vi "Ref Plots Viewer.vi"() -> ()   [LabVIEW 2020]
uses:
  Typedefs/Ref plot graphs cluster.ctl
  RIG-SPECIFIC FILES/FPGA Refs/FPGA Ref.ctl
  Movement Correction/Typedefs/Reference plots window ctrl refs.ctl
  Typedefs/Save-Load enum.ctl
  Typedefs/Read Write Enum.ctl
  Global Variables/General Globals.vi
  Globals/gl_Windows Ctrl refs.vi
  <vilib>/Utility/error.llb/Error Cluster From Error Code.vi
  <vilib>/rvi/errors/niLvFpgaAdjustHostInterfaceError.vi
  <vilib>/rvi/interface/nirviReadWriteControl/nirviReadWriteControl.xnode
  <vilib>/rvi/interface/Simulation/niFpgaSimulationCallBeginRW.vi
  NiFpgaLv.dll
panel:
  out "Test GraphData Path":path
  in  "Append Date-Time":bool
  in  "Append file name":string
  out "MC Data Save ON":bool
  in  "Save MC Data":bool
  in  "Nth Frame":u16=11 min=10 step=10
  out "seen start":i16(graph)
  out "stop_bg":i16(graph)
  out "go_to_bg":i16(graph)
  out "MC":i16(graph)
  out "live_scan ind":i16(graph)
  out "start int":i16(graph)
  out "end of trial":i16(graph)
  out "bg mc Chart":i16(graph)
  in  "Frames":i16=1
  out "FPGA VI Reference Out":T1
  in  "Maximum Value":i32=4095
  in  "Minimum Value":i32
  out "Ref Image":T2(plugin-control)
  out "background_mc":bool
  out "bgsm_state":T3(ring)
  out "Acquire MC BG":bool
  out "rec_on_bg":bool
  out "aq state":T4(ring)
  in  "timed out?":bool
  in  "Acquisition completed":bool
  out "Protocol":string=" Last imaging type: None"
  out "Stop (ind)":bool
  out "error":errorcluster
  in  "Snapshot file path":path caption="Snapshot file path (data is appended if same file used)"
  in  "Buffer Size":i32=5000 min=5 max=10000 step=100
  in  "Refresh rate (ms)":u32=500 min=10 step=10
  in  "Snapshot":bool
  in  "Reset Graphs":bool
  out "Graphs cluster":T5
  # "(during live imaging)"
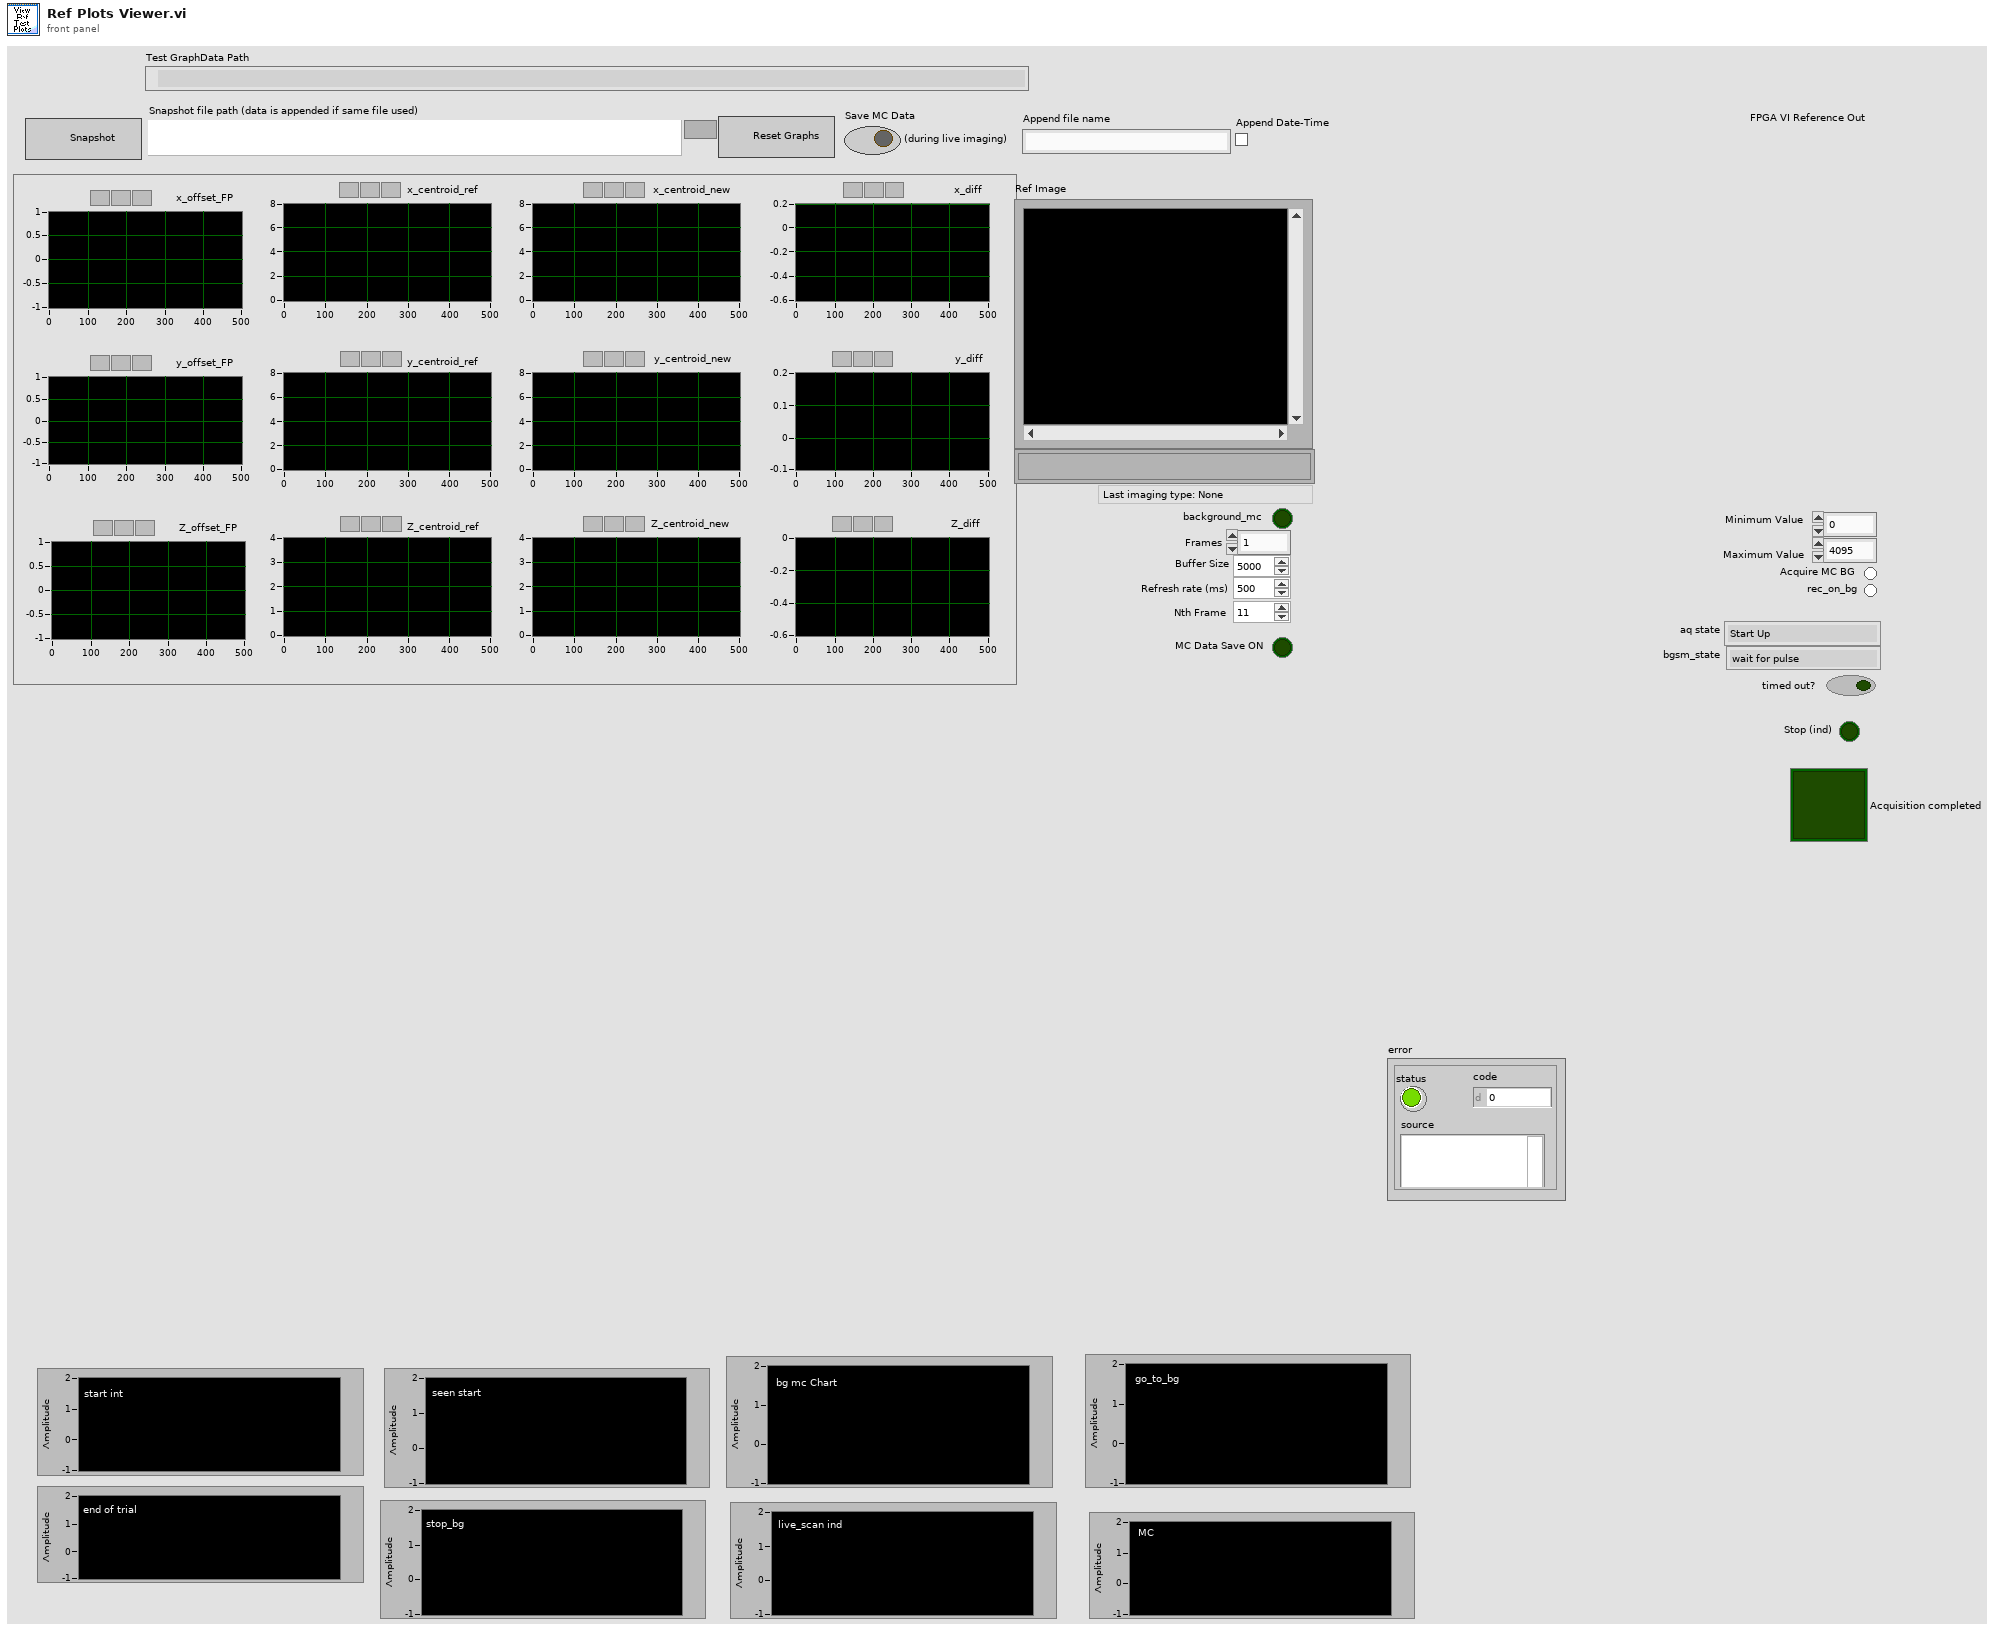
[diagram p1: front panel]
types:
  T1 = typedef "FPGA Ref.ctl" = refnum<k20>
  T2 = typedef "IMAQ Image.ctl" = refnum<image>
  T3 = enum16{"wait for pulse", "wiat for N after pulse", "refernce frame", "ref aod fill bg"}
  T4 = enum16{"Start Up", "Wait for Trigger", "Wait N after Trigger", "DAQ Pointing", "DAQ Scan", "Reference Scan", "Pointing AOL Fill", "Scan AOL FILL", "Reference AOL Fill"}
  T5 = typedef "Ref plot graphs cluster.ctl" = cluster{"x_offset_FP":dbl[], "y_offset_FP":dbl[], "x_centroid_ref":dbl[], "y_centroid_ref":dbl[], "x_centroid_new":dbl[], "y_centroid_new":dbl[], "x_diff":dbl[], "y_diff":dbl[], "Z_offset_FP":dbl[], "Z_centroid_ref":dbl[], "Z_centroid_new":dbl[], "Z_diff":dbl[]}
  T6 = typedef "Image Type" = u32
  T7 = typedef "Reference plots window ctrl refs.ctl" = cluster{"Refresh rate (ms)":refnum<vi>, "Buffer Size":refnum<vi>}
  T8 = typedef "Save-Load enum.ctl" = enum16{"Save to file", "Load from file", "Compare from file", "Save Backup"}
  T9 = enum16{"Obtain queue", "Call window", "Call & send signal", "Release queue"}
  T10 = typedef "Read Write Enum.ctl" = enum16{"Read", "Write"}
  T11 = typedef "AOL_Globals.ctl" = cluster{"Imaging Protocol":T12, "Number of POI":u16, "Number of Miniscans":u16, "Number of Trials":u16, "Number of Cycles ":u64, "# Averaged Frames":u16, "Laser power (%)":u8, "Pockels (V)":dbl, "Acquisition Length (sec)":dbl, "Fill time (us)":dbl, "POI Dwell time (us)":dbl, "Miniscan Dwell time per pixel (us)":dbl, "PMT 1":dbl, "PMT 2":dbl, "Back Apperture (mA)":dbl, "Frame Size":T13, "Center Frequency":dbl, "Field of View (norm)":dbl, "DwellTime (us)":dbl, "Wavelength (nm)":dbl, "Zoom":dbl, "AOL Z":dbl, "AOL Mode":T14, "GridXY":dbl, "GridZ":dbl, "TriggerPeriod (sec)":dbl, "Number of Pixels in Miniscan":u16, "Experiment folder path":path, "X centre":dbl, "Y centre":dbl, "Angle (degrees)":dbl, "Plane Mode":T15, "Threshold":u16[], "Regenerate Chirps":bool, "Rectangle ROI length (pixels)":u16, "Rectangle ROI height (pixels)":u16, "AOD fill":u16, "StartupDelay":i32, "Samples Wait after Trigger":u16, "Slip Cycle":u32, "Add Cycle":bool, "Functional Mode":T16, "Z Start":dbl, "Z Stop":dbl, "# Planes":i32, "Total Pixels":i32, "Variable Miniscan Pixels":u16[], "Use Variable Length":bool, "Use Variable Resolution":bool, "Laser power (%) at Z Start":u8, "Laser power (%) at Z Stop":u8, "Ref Z Step":i8, "Ref Dwell Time (us)":dbl, "Field of View (um)":dbl}
  T12 = typedef "Imaging Protocols enum.ctl" = enum16{"AOL Z-Stack", "Motor Z Stack", "Functional Acquisition", "Single Plane Acquisition", "Volume Acquisition", "Live Imaging", "Live Plane Imaging", "Live Volume Imaging"}
  T13 = typedef "Frame Size.ctl" = u16
  T14 = typedef "AOL modes.ctl" = enum16{"Raster", "Structural", "Pointing", "Mini Scan", "Alignment"}
  T15 = typedef "Plane Mode.ctl" = u16
  T16 = typedef "Functional Mode.ctl" = enum16{"Point", "Line", "Patch", "Plane", "Volume"}
  T17 = enum16{"Start Up", "Wait for Trigger", "Wait N after Trigger", "DAQ Pointing", "DAQ Scan", "Reference Scan", "Pointing AOL Fill", "Scan AOL FILL", "Reference AOL Fill", "galvo_moving"}
  T18 = cluster{"Conversion Method":u32, "Minimum Value":i32, "Maximum Value":i32, "Number Of Shifts":i32}
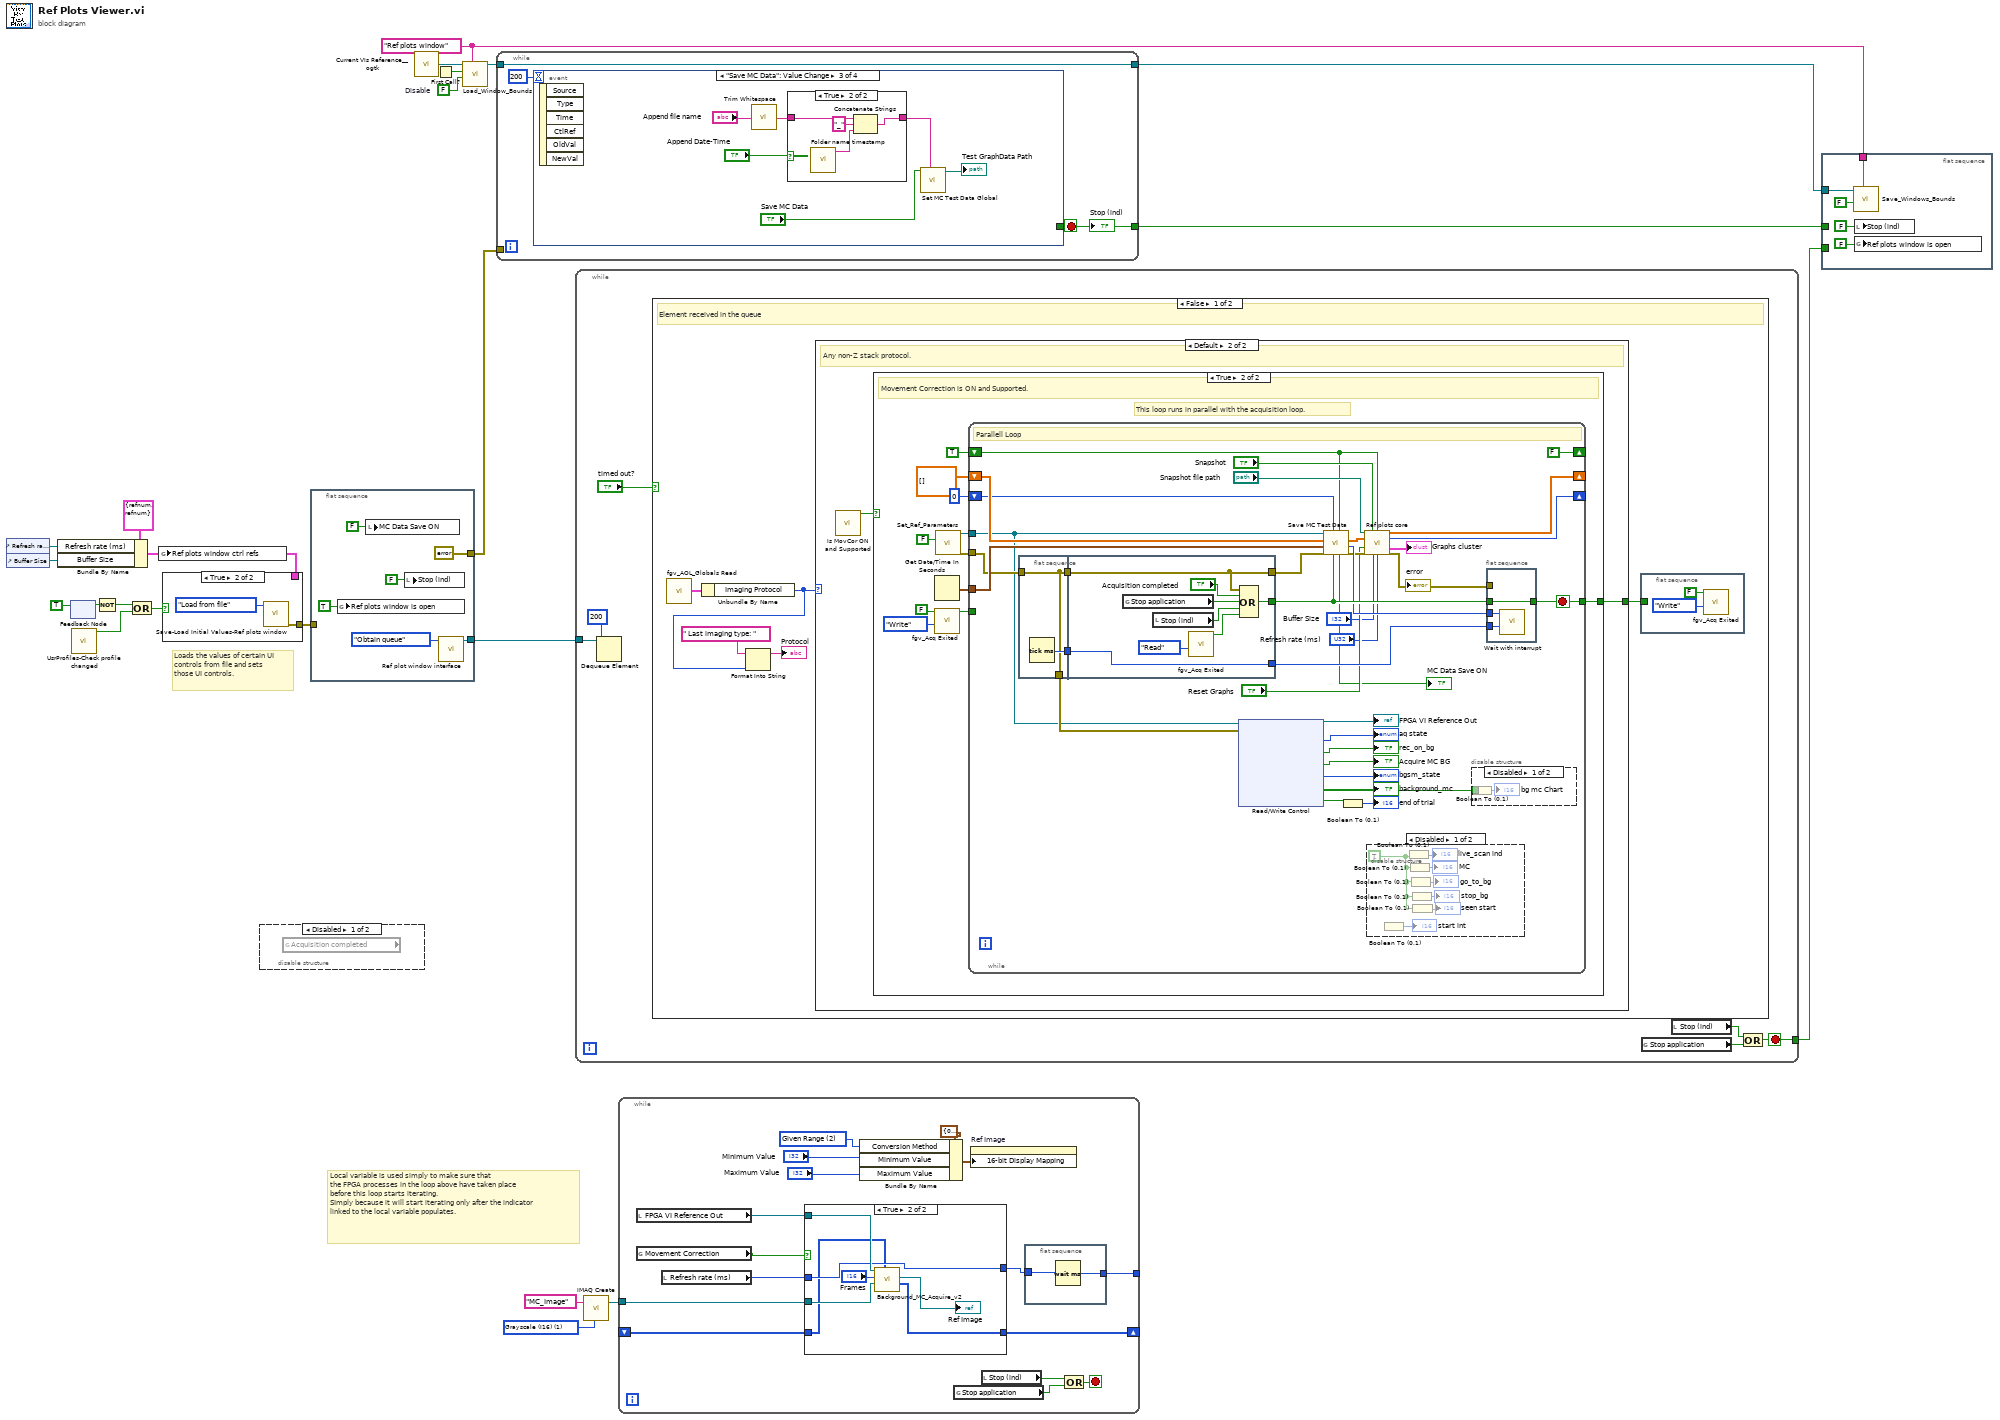
[diagram p0: block diagram]
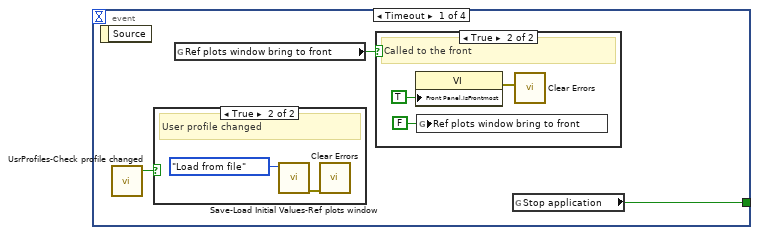
[diagram p5: hidden frame]
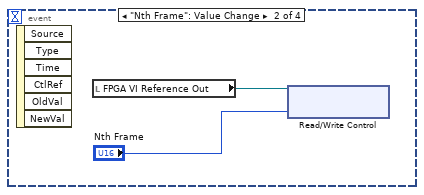
[diagram p8: hidden frame]
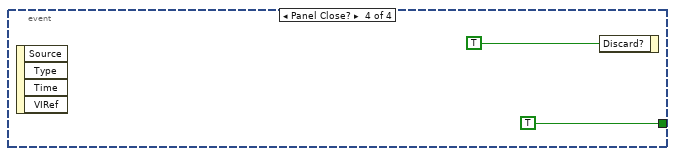
[diagram p10: hidden frame]
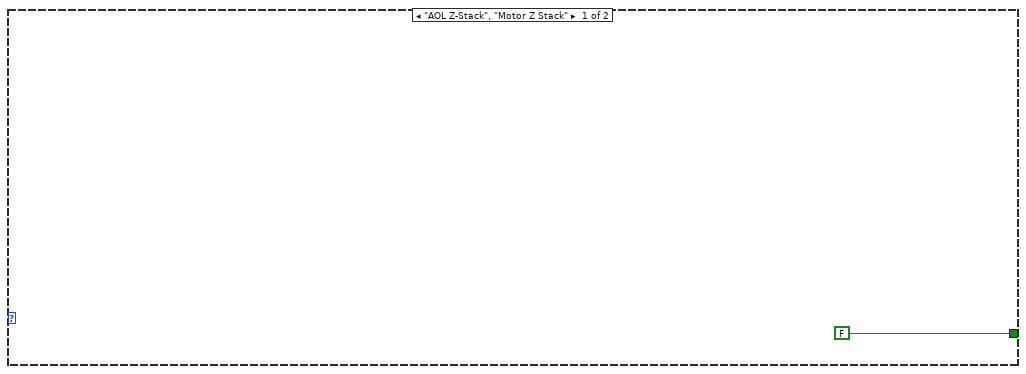
[diagram p11: hidden frame]
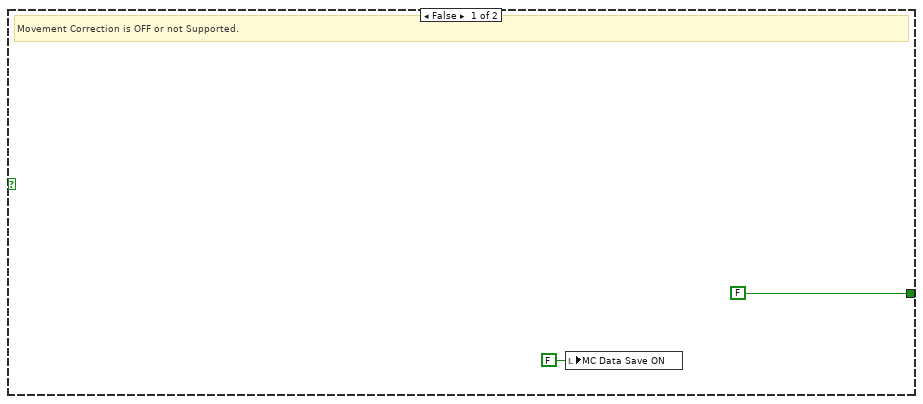
[diagram p12: hidden frame]
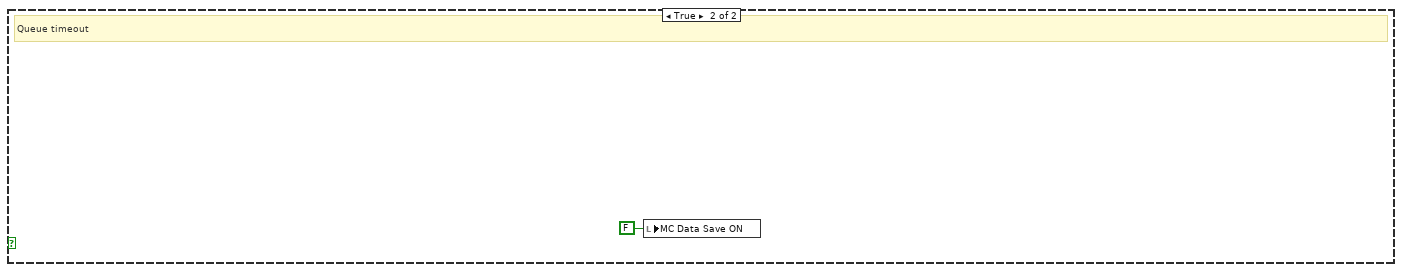
[diagram p15: hidden frame]
diagram:
  w2 = T6 1 items=["Grayscale (U8)", "Grayscale (I16)", "Grayscale (SGL)", "Complex (CSG)", "RGB (U32)", "HSL (U32)", "RGB (U64)", "Grayscale (U16)"] ("Image Type")
  w18 = FALSE  # Disable
  w6 = "Ref plots window" ("Window Name (i.e. Key)")
  # "Local variable is used simply to make sure that\nthe FPGA processes in the loop above have taken place\nbefore this loop starts iterating.\nSImply because it will start iterating only after the indicator\nlinked to the local variable populates."
  # "Loads the values of certain UI controls from file and sets those UI controls."
  n1 = control-ref of="Refresh rate (ms)"() -> (w13:refnum<vi>)
  n2 = control-ref of="Buffer Size"() -> (w12:refnum<vi>)
  n3 = Bundle By Name(cluster=T7 {"Refresh rate (ms)"=refnum, "Buffer Size"=refnum} ("Reference plots window ctrl refs"), "Refresh rate (ms)"=w13, "Buffer Size"=w12) -> (w14:T7)
  n4 = feedback #1() -> (w11:bool)  [unwired: 1 in]
  n5 = feedback-in #1(TRUE) -> ()
  n6 = call "UsrProfiles-Check profile changed.vi"() -> ("Profile changed"=w8:bool)  [unwired: 10 in, 1 out]
  n7 = Not(x=w11) -> (.not. x?=w9:bool)
  n8 = Compound Arithmetic op=OR(w9, w8) -> (w7:bool)
  n9 = global write "gl_Windows Ctrl refs.vi" "Ref plots window ctrl refs"(w14) -> ()
  n10 = case shown="True" w7 {
    tunnel: [_ w24] -> w16
    tunnel: w14 -> [_ _]
    frame False {
    }
    frame True {
      n11 = call "Save-Load Initial Values-Ref plots window.vi"("Function"=Save-Load_enum."Load from file") -> ("error out"=w24:errorcluster)  [unwired: 10 in]
    }
  }
  n12 = disable-structure shown="Disabled" {
    frame Disabled {
      n13 = global read "General Globals.vi" "Acquisition completed"() -> ()  [unwired: 1 out]
    }
    frame Enabled {
    }
  }
  n14 = flat-sequence {
    tunnel: [w30] -> w23
    tunnel: [errorcluster {"status"=FALSE, "code"=0, "source"=""} ("error out")] -> w21
    tunnel: w16 -> [_]
    frame #0 {
      n15 = global write "General Globals.vi" "Ref plots window is open"(TRUE ("Ref plots window is open")) -> ()
      n16 = local write "MC Data Save ON"(FALSE ("MC Data Save ON")) -> ()
      n17 = local write "Stop (ind)"(FALSE ("Stop (ind)")) -> ()
      n18 = call "Ref plot window interface.vi"("Function"=T9."Obtain queue") -> ("Ref plots window queue"=w30:refnum<queue>)  [unwired: 9 in, 1 out]
    }
  }
  n19 = call <userlib>:"Current VIs Reference__ogtk.vi"() -> ("Current VI's reference"=w20:refnum<vi>)  [unwired: 5 in]
  n20 = First Call?() -> (First Call?: T/F=w19:bool)
  n21 = call "Load_Window_Bounds.vi"("Window Name (i.e. Key)"=w6, "Disable"=w18, "First Call"=w19, "Window VI's Ref"=w20) -> ("reference out"=w17:refnum<vi>)  [unwired: 4 in, 3 out]
  n22 = while {
    tunnel: [w32] -> w4
    tunnel: w21 -> [_]
    tunnel: w17 -> [w33]
    tunnel: [w33] -> w5
    stop <- w32 stop-if-true
    n23 = event shown="[2] \"Save MC Data\": Value Change" {
      selector: _ -> [_ _ _ _]
      dyn-events: _ -> [_ _ _ _]
      timeout: 200 -> [_ _ _ _]
      tunnel: [w37 _ _ TRUE ("Stop application")] -> w32
      event Timeout {
        n24 = event-data() -> ()  [unwired: 1 in, 1 out]
        n25 = call "UsrProfiles-Check profile changed.vi"() -> ("Profile changed"=w35:bool)  [unwired: 10 in, 1 out]
        n26 = case shown="True" w35 {
          frame False {
            # "Idle"
          }
          frame True {
            # "User profile changed"
            n27 = call "Save-Load Initial Values-Ref plots window.vi"("Function"=Save-Load_enum."Load from file") -> ("error out"=w38:errorcluster)  [unwired: 10 in]
            n28 = call <vilib>:"Clear Errors.vi"("error in (no error)"=w38) -> ()  [unwired: 5 in, 2 out]
          }
        }
        n29 = global read "General Globals.vi" "Ref plots window bring to front"() -> (w36:bool)
        n30 = case shown="True" w36 {
          frame False {
            # "Idle"
          }
          frame True {
            # "Called to the front"
            n31 = property class="VI"("Front Panel.IsFrontmost"=TRUE ("Front Panel Window:Is Frontmost")) -> (error out=w41:errorcluster)  [unwired: 2 in, 1 out]
            n32 = global write "General Globals.vi" "Ref plots window bring to front"(FALSE ("\"Funct img\" bring to front")) -> ()
            n33 = call <vilib>:"Clear Errors.vi"("error in (no error)"=w41) -> ()  [unwired: 5 in, 2 out]
          }
        }
        n34 = global read "General Globals.vi" "Stop application"() -> (w37:bool)
      }
      event "Nth Frame": Value Change {
        n35 = event-data() -> ()  [unwired: 1 in, 6 out]
        n36 = local read "FPGA VI Reference Out"() -> (w44:T1)
        n37 = xnode "Read/Write Control"("FPGA VI Reference In"=w44, "ref_frame dilute"="Nth Frame") -> ()  [unwired: 1 in, 2 out]
      }
      event "Save MC Data": Value Change {
        n38 = event-data() -> ()  [unwired: 1 in, 6 out]
        n39 = call <vilib>:"Trim Whitespace.vi"("string"="Append file name") -> ("trimmed string"=w48:string)  [unwired: 1 in]
        n40 = case shown="True" "Append Date-Time" {
          tunnel: w48 -> [w51 w55]
          tunnel: [w51 w52] -> w47
          frame False {
          }
          frame True {
            n41 = call "Folder name timestamp.vi"() -> ("date/time string"=w53:string)  [unwired: 11 in]
            n42 = Concatenate Strings(w55, "_" ("string"), w53) -> (w52:string)
          }
        }
        n43 = call "Set MC Test Data Global.vi"("Append Name"=w47, "Save MC TestData"="Save MC Data") -> ("Test GraphData Path"=→"Test GraphData Path":path)  [unwired: 8 in, 1 out]
      }
      event Panel Close? {
        n44 = event-data() -> ()  [unwired: 1 in, 4 out]
        n45 = event-data("Discard?"=TRUE) -> ()  [unwired: 1 in, 1 out]
      }
    }
    "Stop (ind)" <- w32
  }
  n46 = while {
    tunnel: [w60] -> w22
    tunnel: w23 -> [w62]
    stop <- w60 stop-if-true
    n47 = Dequeue Element(queue=w62, timeout in ms (-1)=200) -> ()  [unwired: 1 in, 4 out]
    n48 = case shown="False" "timed out?" {
      frame False {
        # "Element received in the queue"
        n49 = call "fgv_AOL_Globals Read.vi"() -> ("AOL_Globals"=w67:T11)  [unwired: 9 in, 2 out]
        n50 = Unbundle By Name(w67) -> ("Imaging Protocol"=w66:T12)
        n51 = Format Into String(initial string=" Last imaging type: ", w66) -> (resulting string=→"Protocol":string)  [unwired: 2 in, 1 out]
        n52 = case shown="Default" w66 {
          tunnel: [FALSE w71] -> w68
          frame "AOL Z-Stack", "Motor Z Stack" {
          }
          frame Default {
            # "Any non-Z stack protocol."
            n53 = call "Is MovCor ON and Supported.vi"() -> ("MovCor is ON and Supported"=w70:bool)  [unwired: 11 in]
            n54 = case shown="True" w70 {
              tunnel: [FALSE w78] -> w71
              frame False {
                # "Movement Correction is OFF or not Supported."
                n55 = local write "MC Data Save ON"(FALSE ("MC Data Save ON")) -> ()
              }
              frame True {
                # "This loop runs in parallel with the acquisition loop."
                # "Movement Correction is ON and Supported."
                n56 = Get Date/Time In Seconds() -> (seconds since 1Jan1904=w80:timestamp)
                n57 = call "fgv_Acq Exited.vi"("Function"=Read_Write_Enum."Write", "Acquisition completed"=FALSE ("Timelapse?")) -> ("Acquisition completed"=w76:bool)  [unwired: 8 in, 1 out]
                n58 = call "Set_Ref_Parameters.vi"("use_increment_halfrate"=FALSE) -> ("error out"=w82:errorcluster, "FPGA VI Reference Out"=w81:T1)  [unwired: 8 in, 1 out]
                n59 = while {
                  tunnel: w81 -> [w90]
                  tunnel: w82 -> [w111]
                  shift-right: [w107] -> _
                  shift-left: dbl[][] [] -> [w117]
                  tunnel: w80 -> [w118]
                  shift-right: [FALSE] -> _
                  shift-left: TRUE -> [w96]
                  tunnel: [w116] -> w78
                  tunnel: w76 -> [_]
                  shift-right: [w106] -> _
                  shift-left: u32 0 ("Actual refresh rate (ms)") -> [w115]
                  stop <- w116 stop-if-true
                  # "Parallell Loop"
                  n60 = flat-sequence {
                    tunnel: [w130] -> w113
                    tunnel: [w129] -> w112
                    tunnel: w111 -> [w129]
                    tunnel: [w129] -> w91
                    tunnel: [w136] -> w109
                    tunnel: [w135] -> w114
                    tunnel: w113 -> [w135]
                    tunnel: w112 -> [w134]
                    tunnel: [w134] -> w110
                    frame #0 {
                      n61 = Tick Count (ms)() -> (millisecond timer value=w130:u32)
                    }
                    frame #1 {
                      n62 = global read "General Globals.vi" "Stop application"() -> (w138:bool)
                      n63 = local read "Stop (ind)"() -> (w132:bool)
                      n64 = call "fgv_Acq Exited.vi"("Function"=Read_Write_Enum."Read") -> ("Acquisition completed"=w133:bool)  [unwired: 9 in, 1 out]
                      n65 = Compound Arithmetic op=OR(w134, "Acquisition completed", w138, w132, w133) -> (w136:bool)
                    }
                  }
                  n66 = xnode ("Read/Write Control")("FPGA VI Reference In"=w90, "error in"=w91) -> ("FPGA VI Reference Out"=→"FPGA VI Reference Out":T1, "aq state"=→"aq state":T17, "rec_on_bg"=→"rec_on_bg":bool, "Acquire MC BG"=→"Acquire MC BG":bool, "bgsm_state"=→"bgsm_state":T3, "background_mc"=w88:bool, "end of trial"=w86:bool)  [unwired: 1 out]
                  "background_mc" <- w88
                  n67 = call "Save MC Test Data.vi"("Initialise"=w96, "Stop"=w109, "Actual refresh rate (ms)"=w115, "error in (no error)"=w110, "Initial Time Stamp"=w118, "Test Data In"=w117, "FPGA Ref in"=w90) -> ("error out"=w104:errorcluster, "MC state"=w108:enum16{"Waiting", "First frame", "Wrote Ref"}, "Test Data Out"=w97:dbl[][], "MC Data Save ON"=→"MC Data Save ON":bool)  [unwired: 1 in]
                  n68 = Boolean To (0,1)(Boolean=w86) -> (0, 1=→"end of trial":i16)
                  n69 = call "Ref plots core.vi"("Snapshot file path"="Snapshot file path", "Snapshot"="Snapshot", "Initialise"=w96, "Ref Test Data in in"=w97, "Reset Graphs"="Reset Graphs", "error in (no error)"=w104, "Buffer Size"="Buffer Size", "Refresh rate (ms)"="Refresh rate (ms)") -> ("Ref Test Data out"=w107:dbl[][], "Actual refresh rate (ms)"=w106:u32, "Graphs cluster"=→"Graphs cluster":T5, "error"=w105:errorcluster)  [unwired: 4 in]
                  "error" <- w105
                  n70 = disable-structure shown="Disabled" {
                    frame Disabled {
                      w121 = TRUE
                      n71 = Boolean To (0,1)() -> (0, 1=→"start int":i16)  [unwired: 1 in]
                      n72 = Boolean To (0,1)(Boolean=w121) -> (0, 1=→"live_scan ind":i16)
                      n73 = Boolean To (0,1)(Boolean=w121) -> (0, 1=→"MC":i16)
                      n74 = Boolean To (0,1)(Boolean=w121) -> (0, 1=→"go_to_bg":i16)
                      n75 = Boolean To (0,1)(Boolean=w121) -> (0, 1=→"stop_bg":i16)
                      n76 = Boolean To (0,1)(Boolean=w121) -> (0, 1=→"seen start":i16)
                    }
                    frame Enabled {
                    }
                  }
                  n77 = disable-structure shown="Disabled" {
                    disable-tunnel: w88 -> [w128 _]
                    frame Disabled {
                      n78 = Boolean To (0,1)(Boolean=w128) -> (0, 1=→"bg mc Chart":i16)
                    }
                    frame Enabled {
                    }
                  }
                  n79 = flat-sequence {
                    tunnel: w109 -> [w141]
                    tunnel: [w141] -> w116
                    tunnel: w114 -> [w140]
                    tunnel: w108 -> [w139]
                    tunnel: w105 -> [_]
                    frame #0 {
                      n80 = call "Wait with interrupt.vi"("Tick count at loop start (ms)"=w140, "Loop iteration (ms)"=w139) -> ()  [unwired: 10 in]
                    }
                  }
                }
              }
            }
          }
        }
        n81 = flat-sequence {
          tunnel: w68 -> [_]
          frame #0 {
            n82 = call "fgv_Acq Exited.vi"("Function"=Read_Write_Enum."Write", "Acquisition completed"=FALSE ("Timelapse?")) -> ()  [unwired: 8 in, 2 out]
          }
        }
      }
      frame True {
        # "Queue timeout"
        n83 = local write "MC Data Save ON"(FALSE ("MC Data Save ON")) -> ()
      }
    }
    n84 = global read "General Globals.vi" "Stop application"() -> (w63:bool)
    n85 = local read "Stop (ind)"() -> (w59:bool)
    n86 = Compound Arithmetic op=OR(w59, w63) -> (w60:bool)
  }
  n87 = call "IMAQ Create"("Image Name"="MC_Image", "Image Type"=w2) -> ("New Image"=w1:T2)  [unwired: 3 in, 1 out]
  n88 = while {
    tunnel: w1 -> [w157]
    tunnel: [w148] -> _
    shift-right: [w146] -> _
    shift-left: _ -> [w145]
    stop <- w158 stop-if-true
    w150 = u32 2 items=["Full Dynamic", "Downshift", "Given Range", "90% Dynamic", "Given Percent Range"] ("Conversion Method (Given Range)")
    n89 = local read "FPGA VI Reference Out"() -> (w156:T1)
    n90 = global read "General Globals.vi" "Movement Correction"() -> (w147:bool)
    n91 = local read "Refresh rate (ms)"() -> (w155:u32)
    n92 = case shown="True" w147 {
      tunnel: w156 -> [_ w171]
      tunnel: w157 -> [_ w170]
      tunnel: w155 -> [w164 w167]
      tunnel: [w164 w167] -> w149
      tunnel: [w163 w166] -> w146
      tunnel: w145 -> [w163 w165]
      frame False {
      }
      frame True {
        n93 = call "Background_MC_Acquire_v2.vi"("prev deleted portion"=w165, "Image In"=w170, "Frames"="Frames", "FPGA VI Reference In"=w171) -> ("deleted portion"=w166:u16[], "Image"=→"Ref Image":T2)  [unwired: 4 in, 2 out]
      }
    }
    n94 = Bundle By Name(cluster=T18 {"Conversion Method"=0, "Minimum Value"=0, "Maximum Value"=0, "Number Of Shifts"=0} ("16-bit Display Mapping:All Elements"), "Conversion Method"=w150, "Minimum Value"="Minimum Value", "Maximum Value"="Maximum Value") -> (w152:T18)
    n95 = global read "General Globals.vi" "Stop application"() -> (w159:bool)
    n96 = property on="Ref Image" class="ImageControl"("16-bit Display Mapping"=w152) -> ()  [unwired: 2 in, 2 out]
    n97 = local read "Stop (ind)"() -> (w160:bool)
    n98 = flat-sequence {
      tunnel: [w162] -> w148
      tunnel: w149 -> [w161]
      frame #0 {
        n99 = Wait (ms)(milliseconds to wait=w161) -> (millisecond timer value=w162:u32)
      }
    }
    n100 = Compound Arithmetic op=OR(w160, w159) -> (w158:bool)
  }
  n101 = flat-sequence {
    tunnel: w22 -> [_]
    tunnel: w6 -> [w173]
    tunnel: w5 -> [w172]
    tunnel: w4 -> [_]
    frame #0 {
      n102 = call "Save_Windows_Bounds.vi"("Window Name (i.e. Key)"=w173, "Front Panel Window:Open"=FALSE, "Window VI's Ref"=w172) -> ()  [unwired: 8 in, 1 out]
      n103 = local write "Stop (ind)"(FALSE ("Stop (ind)")) -> ()
      n104 = global write "General Globals.vi" "Ref plots window is open"(FALSE ("Ref plots window is open")) -> ()
    }
  }
